vi "_tmp2.vi"() -> ()   [LabVIEW 2019]
uses:
  lib/Element Type.ctl
  lib/Element.ctl
  lib/labview_json.lvlib
panel:
  out "error out":errorcluster
  in  "JSON Path":string[](array[string])
  out "JSON":string
  # "c,1 == {\"c\":[null,true]}"
  # "1 = Array([null, X])\nc = Object("
  # "d = {a:1,b:2}\n\nd[a]"
  # "a.b.c = {\"a\":{\"b\":{\"c\":VALUE}}}"
  # "a.b.0 = {\"a\":{\"b\":[VALUE]}}"
  # "a.0.b = {\"a\":[{\"b\":VALUE}]}"
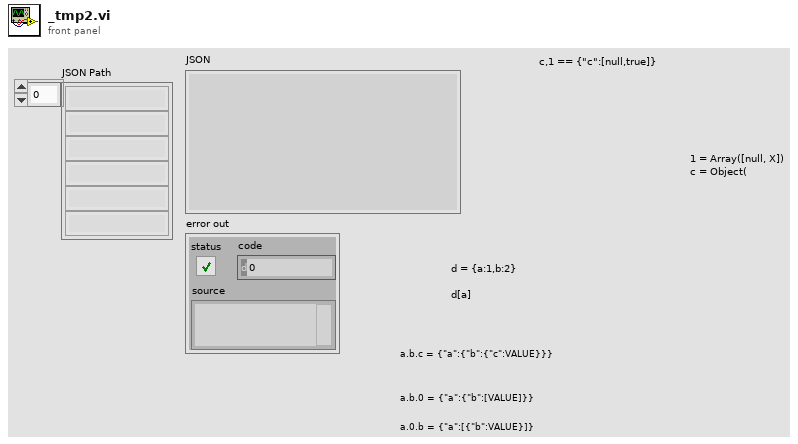
[diagram p1: front panel]
types:
  T1 = typedef "labview_json.lvlib/Element.ctl" = cluster{"Key":string, "Type":T2, "Value":variant}
  T2 = typedef "labview_json.lvlib/Element Type.ctl" = enum8{"NULL", "OBJECT", "ARRAY", "BOOL", "INT", "UINT", "FLOAT", "STRING"}
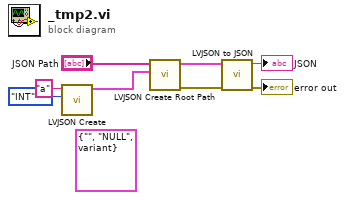
[diagram p0: block diagram]
diagram:
  (unwired) T1 {"Key"="", "Type"=enum."NULL", "Value"=variant} ("Value in")
  n1 = call "LVJSON Create.vi"("Type"=Element_Type."INT", "Key"="a") -> ("Element out"=w1:T1)  [unwired: 9 in]
  n2 = call "LVJSON Create Root Path.vi"("Element in"=w1, "Root Path"="JSON Path") -> ("error out"=w7:errorcluster, "Root Element out"=w8:T1)  [unwired: 8 in]
  n3 = call "LVJSON to JSON.vi"("error in (no error)"=w7, "Root Element in"=w8) -> ("error out"=→"error out":errorcluster, "JSON out"=→"JSON":string)  [unwired: 7 in, 1 out]
